vi "KE2657A_Test.vi"(8 "error in (no error)":errorcluster, 11 "KE2657A.lvclass":refnum<class "KE2657A.lvclass">) -> (0 "error out":errorcluster, 3 "KE2657A out":refnum<class "KE2657A.lvclass">)   [LabVIEW 2018, in "KE2657A.lvclass"]
uses:
  KE2657A.lvclass
  <vilib>/Platform/TimedLoop/XDataNode/timing_clust.ctl
  <vilib>/Platform/TimedLoop/XDataNode/nitl_modes.ctl
  <vilib>/Platform/TimedLoop/XDataNode/wakeup.ctl
  InstrumentSetup.vi
  <vilib>/platform/TimedLoop/XDataNode/XDataNode.xnode
  <vilib>/Platform/TimedLoop/XDataNode/XDNodeRunTimeDep.lvlib
  InstrControl.lvclass
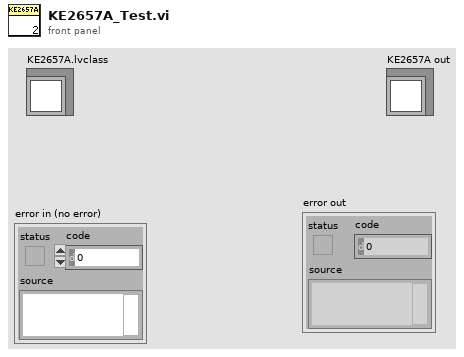
[diagram p1: front panel]
types:
  T1 = cluster{"KE 2410":cluster{"Instrument name":string, "address":refnum<visa-resource-name>, "Instrument type":u16}, "KE 6517":cluster{"Instrument name":string, "address":refnum<visa-resource-name>, "Instrument type":u16}, "KE 487":cluster{"Instrument name":string, "address":refnum<visa-resource-name>, "Instrument type":u16}, "KE 236":cluster{"Instrument name":string, "address":refnum<visa-resource-name>, "Instrument type":u16}, "WK 6440B":cluster{"Instrument name":string, "address":refnum<visa-resource-name>, "Instrument type":u16}, "WK 6425":cluster{"Instrument name":string, "address":refnum<visa-resource-name>, "Instrument type":u16}, "Pickering Matrix":cluster{"Instrument name":string, "address":refnum<visa-resource-name>, "Instrument type":u16}, "KE 2000":cluster{"Instrument name":string, "address":refnum<visa-resource-name>, "Instrument type":u16}, "KE3706A Switching":cluster{"Instrument name":string, "address":refnum<visa-resource-name>, "Instrument type":u16}, "HP 4284A":cluster{"Instrument name":string, "address":refnum<visa-resource-name>, "Instrument type":u16}, "KE237":cluster{"Instrument name":string, "address":refnum<visa-resource-name>, "Instrument type":u16}, "KE2657A":cluster{"Instrument name":string, "address":refnum<visa-resource-name>, "Instrument type":u16}}
  T2 = cluster{"Compliance [A]":sgl, "Voltage range (source)":enum16{"Auto", "200 V", "500 V", "1500 V", "3000 V"}, "Current range (measure)":enum16{"Auto", "1 nA", "10 nA", "100 nA", "1 uA", "10 uA", "100 uA", "1 mA", "2 mA", "20 mA", "120 mA"}, "KE2657A":refnum<class "KE2657A.lvclass">}
  T3 = typedef "XDNodeRunTimeDep.lvlib/timing_clust.ctl" = cluster{"Expected End [f-1]":u64, "Actual End [f-1]":u64, "Finished Late? [f-1]":bool, "Expected End [i-1]":u64, "Actual End [i-1]":u64, "Finished Late? [i-1]":bool, "Expected Start [i]":u64, "Actual Start [i]":u64, "Expected Start [f]":u64, "Actual Start [f]":u64, "Source Name":string, "Structure Name":string, "Period":i64, "Deadline":i64, "Offset":i64, "Start":i64, "Priority":i32, "Timeout":i32, "Mode":T4, "Wakeup Reason":T5, "Error":errorcluster, "Source Type":string, "Secondary Source Type":string, "Global End Time":u64, "Global Start Time":u64, "Frame Duration":u64, "Iteration Duration":u64, "Assigned CPU":i32, "I/O Scan Engine Mode":u32}
  T4 = typedef "XDNodeRunTimeDep.lvlib/nitl_modes.ctl" = enum32{"No Change", "Process missed periods, maintain original phase", "Discard missed periods, maintain original phase", "Process missed periods, ignore original phase", "Discard missed periods, ignore original phase"}
  T5 = typedef "XDNodeRunTimeDep.lvlib/wakeup.ctl" = enum32{"Normal", "Aborted", "Asynchronous wakeup", "Timing source error", "Timed loop error", "Timeout"}
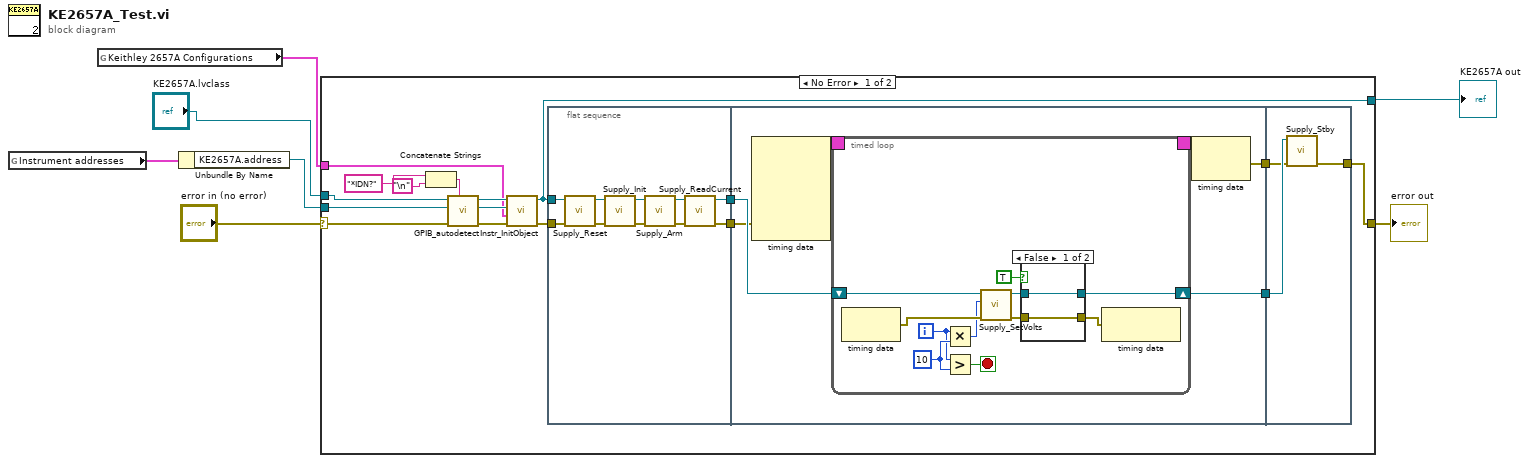
[diagram p0: block diagram]
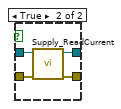
[diagram p2: hidden frame]
diagram:
  n1 = global read "InstrumentSetup.vi" "Instrument addresses"() -> (w5:T1)
  n2 = global read "InstrumentSetup.vi" "Keithley 2657A Configurations"() -> (w3:T2)
  n3 = Unbundle By Name(w5) -> ("KE2657A.address"=w4:refnum<visa-resource-name>)
  n4 = case shown="No Error" "error in (no error)" {
    selector: "error in (no error)" -> [w17 w72]
    tunnel: "KE2657A.lvclass" -> [w14 w71]
    tunnel: [w20 w71] -> w1
    tunnel: [w19 w72] -> w7
    tunnel: w4 -> [w15 _]
    tunnel: w3 -> [w11 _]
    frame No Error {
      n5 = Concatenate Strings("*IDN?" ("regular expression"), "\n") -> (w8:string)
      n6 = call-dynamic "GPIB_autodetect.vi"("ID command"=w8, "error in (no error)"=w17, "Instrument address in"=w15, "InstrControl in"=w14) -> ("error out"=w16:errorcluster, "Instrument address out"=w12:refnum<visa-resource-name>, "InstrControl out"=w13:refnum<class "KE2657A.lvclass">)  [unwired: 5 in]
      n7 = call-dynamic "Instr_InitObject.vi"("error in (no error)"=w16, "Instrument Configuration"=w11, "Instrument address"=w12, "KE2657A in"=w13) -> ("error out"=w21:errorcluster, "KE2657A out"=w20:refnum<class "KE2657A.lvclass">)  [unwired: 6 in]
      n8 = flat-sequence {
        tunnel: w21 -> [w29]
        tunnel: w20 -> [w28]
        tunnel: [w26] -> w24
        tunnel: [w25] -> w18
        tunnel: w24 -> [w40]
        tunnel: [w39] -> w23
        tunnel: [w36] -> w22
        tunnel: w18 -> [w35]
        tunnel: [w68] -> w19
        tunnel: w23 -> [w69]
        tunnel: w22 -> [w70]
        frame #0 {
          n9 = call-dynamic "Supply_Reset.vi"("error in (no error)"=w29, "SupplyControl in"=w28) -> ("error out"=w33:errorcluster, "SupplyControl out"=w27:refnum<class "KE2657A.lvclass">)  [unwired: 8 in]
          n10 = call-dynamic "Supply_Init.vi"("error in (no error)"=w33, "SupplyControl in"=w27) -> ("error out"=w32:errorcluster, "SupplyControl out"=w34:refnum<class "KE2657A.lvclass">)  [unwired: 8 in]
          n11 = call-dynamic "Supply_Arm.vi"("error in (no error)"=w32, "SupplyControl in"=w34) -> ("error out"=w30:errorcluster, "SupplyControl out"=w31:refnum<class "KE2657A.lvclass">)  [unwired: 8 in]
          n12 = call-dynamic "Supply_ReadCurrent.vi"("error in (no error)"=w30, "SupplyControl in"=w31) -> ("error out"=w25:errorcluster, "SupplyControl out"=w26:refnum<class "KE2657A.lvclass">)  [unwired: 7 in, 1 out]
        }
        frame #1 {
          n13 = node-c288(w35) -> (w38:T3)  [unwired: 4 in]
          n14 = timed-loop {
            timing: w38 -> [_]
            timing-out: [_] -> w37
            shift-right: [w43] -> w36
            shift-left: w40 -> [w49]
            i -> [w47]
            stop <- w46 stop-if-true
            w48 = 10
            n15 = node-c288() -> (w51:errorcluster)  [unwired: 1 in]
            n16 = Multiply(x=w47, y=w48) -> (x*y=w50:i32)
            n17 = Greater?(x=w47, y=w48) -> (0:w46:bool)
            n18 = call-dynamic "Supply_SetVolts.vi"("error in (no error)"=w51, "Volts IN [V]"=w50, "KE2657A in"=w49) -> ("error out"=w45:errorcluster, "KE2657A out"=w44:refnum<class "KE2657A.lvclass">)  [unwired: 6 in, 1 out]
            n19 = case shown="False" TRUE {
              tunnel: w45 -> [w53 w57]
              tunnel: w44 -> [w52 w56]
              tunnel: [w52 w55] -> w43
              tunnel: [w53 w54] -> w42
              frame False {
              }
              frame True {
                n20 = call-dynamic "Supply_ReadCurrent.vi"("error in (no error)"=w57, "SupplyControl in"=w56) -> ("error out"=w54:errorcluster, "SupplyControl out"=w55:refnum<class "KE2657A.lvclass">)  [unwired: 7 in, 1 out]
              }
            }
            n21 = node-c288(w42) -> ()  [unwired: 1 out]
          }
          n22 = node-c288(w37) -> (w39:errorcluster)
        }
        frame #2 {
          n23 = call-dynamic "Supply_Stby.vi"("error in (no error)"=w69, "SupplyControl in"=w70) -> ("error out"=w68:errorcluster)  [unwired: 8 in, 1 out]
        }
      }
    }
    frame Error {
    }
  }
  "error out" <- w7
  "KE2657A out" <- w1
